vi "demo.vi"() -> ()   [LabVIEW 2013]
uses:
  Control/Data.ctl
  Control/State.ctl
  Control/Motor.ctl
panel:
  out "Data":T1={"State"=enum."Idle", "Motor"={"#1"=FALSE, "#2"=FALSE, "#3"=FALSE}, "Timer"=30.0}
  in  "Stop":bool
  in  "Start":bool
  in  "停止":bool
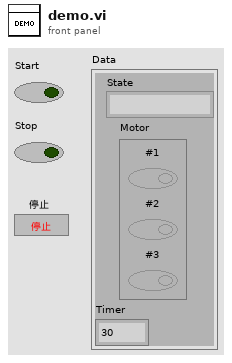
[diagram p1: front panel]
types:
  T1 = typedef "Data.ctl" = cluster{"State":T2, "Motor":T3, "Timer":dbl}
  T2 = typedef "State.ctl" = enum16{"Idle", "#1 Run", "#2 Run", "#3 Run", "#3 Stop", "#2 Stop", "#1 Stop"}
  T3 = typedef "Motor.ctl" = cluster{"#1":bool, "#2":bool, "#3":bool}
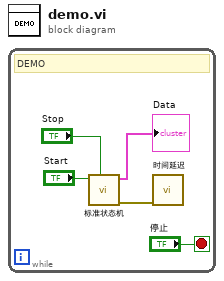
[diagram p0: block diagram]
diagram:
  n1 = while {
    stop <- "停止" stop-if-true
    # "DEMO"
    n2 = call "标准状态机.vi"("Stop"="Stop", "Start"="Start") -> ("error out"=w1:errorcluster, "Status"=→"Data":T1)  [unwired: 8 in]
    n3 = call "时间延迟"("error in (no error)"=w1) -> ()  [unwired: 10 in, 1 out]
  }
